vi "niDTS WLAN UTIL MacString to U64Address.vi"(9 "error in":errorcluster, 10 "Address String":string="00:00:00:00:00:00") -> (1 "error out":errorcluster, 2 "Address U64":u64 format="%x")   [LabVIEW 2014, in "niDTS WLAN.lvlib"]
uses:
  niDTS WLAN.lvlib
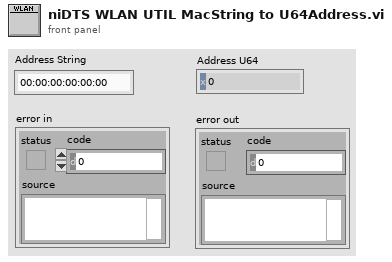
[diagram p1: front panel]
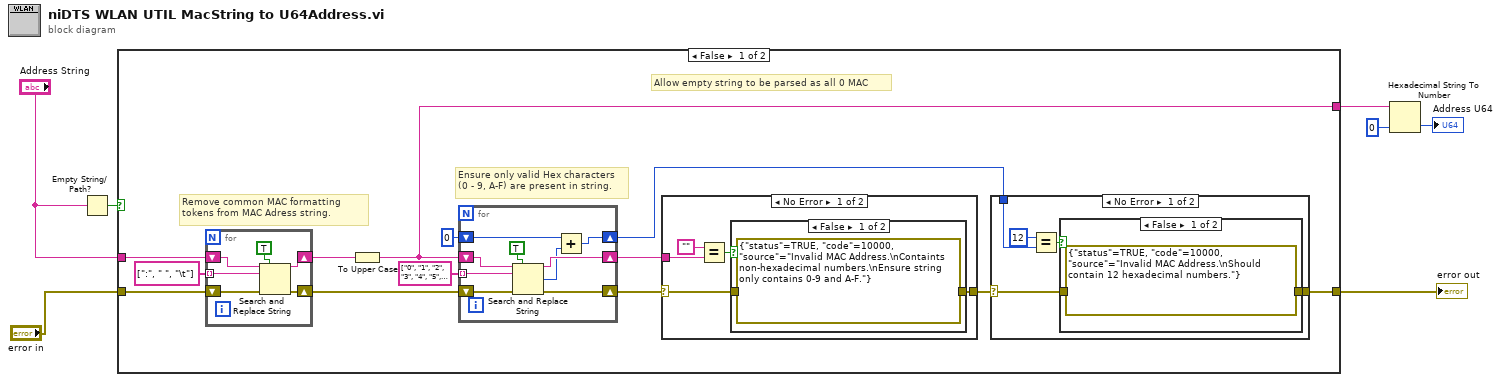
[diagram p0: block diagram]
diagram:
  n1 = Empty String/Path?(string/path="Address String") -> (empty?=w1:bool)
  n2 = case shown="False" w1 {
    tunnel: [w17 w52] -> w5
    tunnel: [w10 w53] -> w4
    tunnel: "error in" -> [w9 w53]
    tunnel: "Address String" -> [w8 w52]
    frame False {
      # "Allow empty string to be parsed as all 0 MAC"
      # "Remove common MAC formatting\ntokens from MAC Adress string."
      # "Ensure only valid Hex characters\n(0 - 9, A-F) are present in string."
      n3 = for {
        tunnel: string[] [":", " ", "\t"] -> [w40] mode=indexing
        shift-right: [w41] -> w14
        shift-left: w8 -> [w42]
        shift-right: [w38] -> w15
        shift-left: w9 -> [w39]
        n4 = Search and Replace String(replace all?=TRUE ("replace all? (F)"), input string=w42, search string=w40, error in=w39) -> (result string=w41:string, error out=w38:errorcluster)  [unwired: 6 out]
      }
      n5 = To Upper Case(1:w14) -> (0:w17:string)
      n6 = for {
        tunnel: string[] ["0", "1", "2", "3", "4", "5", "6", "7", "8", "9", "A", "B", "C", "D", "E", "F"] -> [w49] mode=indexing
        shift-right: [w50] -> w19
        shift-left: w17 -> [w51]
        shift-right: [w47] -> w13
        shift-left: w15 -> [w48]
        shift-right: [w43] -> w11
        shift-left: 0 ("number of replacements") -> [w45]
        n7 = Search and Replace String(replace all?=TRUE ("replace all? (F)"), input string=w51, search string=w49, error in=w48) -> (result string=w50:string, number of replacements=w44:i32, error out=w47:errorcluster)  [unwired: 5 out]
        n8 = Add(x=w45, y=w44) -> (x+y=w43:i32)
      }
      n9 = case shown="No Error" w13 {
        selector: w13 -> [w30 w36]
        tunnel: w19 -> [w33 _]
        tunnel: [w29 w36] -> w12
        frame No Error {
          n10 = Equal?(x="", y=w33) -> (x = y?=w31:bool)
          n11 = case shown="False" w31 {
            tunnel: w30 -> [_ w35]
            tunnel: [errorcluster {"status"=TRUE, "code"=10000, "source"="Invalid MAC Address.\nContaints non-hexadecimal numbers.\nEnsure string only contains 0-9 and A-F."} ("error IO") w35] -> w29
            frame False {
            }
            frame True {
            }
          }
        }
        frame Error {
        }
      }
      n12 = case shown="No Error" w12 {
        selector: w12 -> [w23 w28]
        tunnel: w11 -> [w24 _]
        tunnel: [w21 w28] -> w10
        frame No Error {
          n13 = Equal?(x=12, y=w24) -> (x = y?=w22:bool)
          n14 = case shown="False" w22 {
            tunnel: w23 -> [_ w27]
            tunnel: [errorcluster {"status"=TRUE, "code"=10000, "source"="Invalid MAC Address.\nShould contain 12 hexadecimal numbers."} ("error IO") w27] -> w21
            frame False {
            }
            frame True {
            }
          }
        }
        frame Error {
        }
      }
    }
    frame True {
    }
  }
  "error out" <- w4
  n15 = Hexadecimal String To Number(string=w5, default (0uL)=u64 0 ("default (0 U32)")) -> (number=→"Address U64":u64)  [unwired: 2 out]
